vi "Perform Action.vi"(8 "error in":errorcluster, 10 "Input":variant, 11 "Thermometer DAQmx RTD Cont CFG in":refnum<class "Thermometer DAQmx RTD Cont CFG Simulated.lvclass">) -> (0 "error out":errorcluster, 2 "Output":variant, 3 "Thermometer DAQmx RTD Cont CFG out":refnum<class "Thermometer DAQmx RTD Cont CFG Simulated.lvclass">)   [LabVIEW 2024, in "DAQmx Simulated CFGs.lvlib" / "Thermometer DAQmx RTD Cont CFG Simulated.lvclass"]
uses:
  Thermometer DAQmx RTD Cont CFG Simulated.lvclass
  25f3cd8c-dbf7-49b5-a67b-aca2ec958ed2.vi
  <vilib>/JDP Science/JSONtext/Find Item.vi
  <vilib>/JDP Science/JSONtext/Next JSON Value.vi
  <vilib>/JDP Science/JSONtext/String Subset.vi
  <vilib>/JDP Science/JSONtext/Parsing/Advance past next JSON Value (inlined COPY).vi
  <vilib>/JDP Science/JSONtext/Parsing/Advance past whitespace.vi
  <vilib>/JDP Science/JSONtext/Parsing/Advance past String.vi
  <vilib>/JDP Science/JSONtext/Parsing/Advance past Number.vi
  <vilib>/JDP Science/JSONtext/Parsing/Advance past Line Ending.vi
  <vilib>/JDP Science/JSONtext/Parsing/Parse Full Path or Item Name.vi
  <vilib>/JDP Science/JSONtext/Parsing/Advance past Array.vi
  <vilib>/JDP Science/JSONtext/Parsing/Advance past Object.vi
  <vilib>/JDP Science/JSONtext/support/Error Cluster From Code.vi
  <vilib>/JDP Science/JSONtext/Offset/Find Item Locations by Path.vi
  <vilib>/JDP Science/JSONtext/JSON text to Variant.vi
  <vilib>/JDP Science/JSONtext/LVClass Serializer/JSONtext LVClass Serializer.lvclass
  Thermometer DAQmx RTD Cont CFG/Thermometer DAQmx RTD Cont CFG.lvclass
  Configurations/CFG JSON/CFG JSON.lvclass
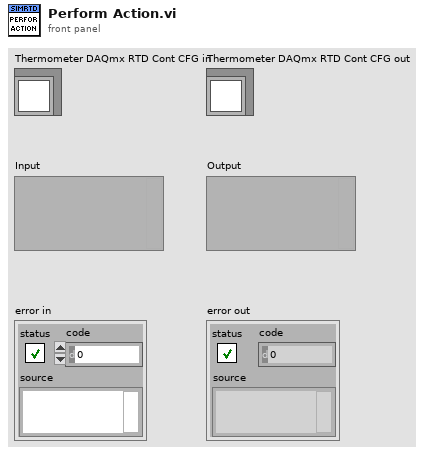
[diagram p1: front panel]
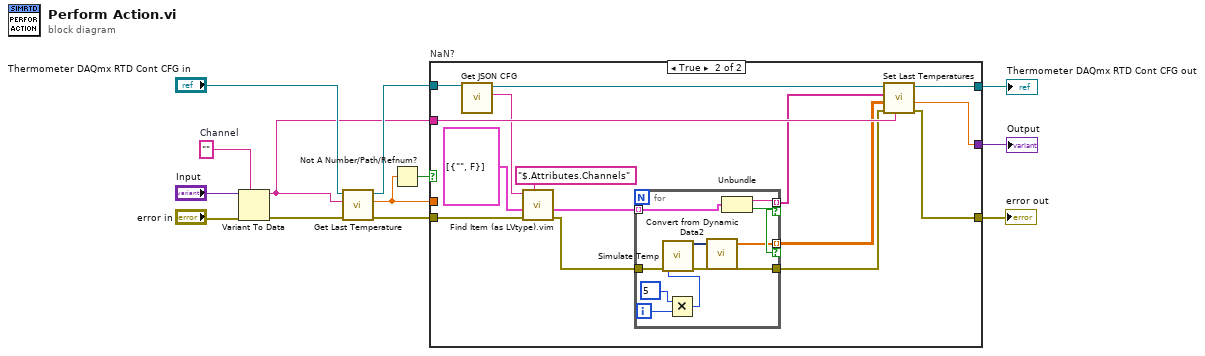
[diagram p0: block diagram]
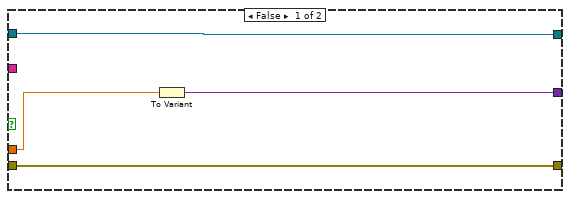
[diagram p2: hidden frame]
diagram:
  w9 = ""  # Channel
  n1 = Variant To Data(error in="error in", type=w9, Variant="Input") -> (data=w1:string, error out=w2:errorcluster)
  n2 = call "Get Last Temperature.vi"("error in"=w2, "Channel"=w1, "Thermometer DAQmx RTD Cont CFG in"="Thermometer DAQmx RTD Cont CFG in") -> ("error out"=w11:errorcluster, "Temperature"=w10:dbl, "Thermometer DAQmx RTD Cont CFG out"=w12:refnum<class "Thermometer DAQmx RTD Cont CFG Simulated.lvclass">)  [unwired: 6 in]
  n3 = Not A Number/Path/Refnum?(number/path/refnum=w10) -> (NaN/Path/Refnum?=w13:bool)
  n4 = case "NaN?" shown="True" w13 {
    tunnel: w12 -> [w15 w28]
    tunnel: w11 -> [w14 w26]
    tunnel: [w14 w32] -> w3
    tunnel: [w16 w29] -> w4
    tunnel: [w15 w31] -> w5
    tunnel: w10 -> [w17 _]
    tunnel: w1 -> [_ w30]
    frame False {
      n5 = To Variant(anything=w17) -> (Variant=w16:variant)
    }
    frame True {
      n6 = call "Get JSON CFG.vi"("CFG JSON in"=w28) -> ("<JSON> CFG"=w27:string, "CFG JSON out"=w21:refnum<class "Thermometer DAQmx RTD Cont CFG Simulated.lvclass">)  [unwired: 9 in]
      n7 = call "Find Item (as LVtype).vim"("$Path or Item Name"="$.Attributes.Channels", "error in (no error)"=w26, "Data Type and Default Value"=cluster{"Name":string, "Enabled":bool}[] [{"Name"="", "Enabled"=FALSE}], "JSON"=w27) -> ("error out"=w20:errorcluster, "Data"=w23:cluster{"Name":string, "Enabled":bool}[])  [unwired: 4 in, 2 out]
      n8 = for {
        tunnel: w23 -> [w42] mode=indexing
        tunnel: [w41] -> w22 mode=indexing if=w38
        tunnel: w20 -> [w40]
        tunnel: [w39] -> w19
        tunnel: [w33] -> w18 mode=indexing if=w38
        i -> [w37]
        n9 = Multiply(x=5, y=w37) -> (x*y=w35:i32)
        n10 = call "Simulate Temp"("Phase"=w35, "error in (no error)"=w40) -> ("Sine Temp 50-60"=w34:dynamicdata, "error out"=w39:errorcluster)  [unwired: 12 in]
        n11 = call "Convert from Dynamic Data2"("Dynamic Data Type"=w34) -> ("Array"=w33:dbl[])  [unwired: 3 in]
        n12 = Unbundle(w42) -> ("Name"=w41:string, "Enabled"=w38:bool)
      }
      n13 = call "Set Last Temperatures.vi"("Read Channel Ident"=w30, "error in"=w19, "Temperatures"=w18, "Channel Idents"=w22, "Thermometer DAQmx RTD Cont CFG in"=w21) -> ("error out"=w32:errorcluster, "Temperature"=w29:dbl, "Thermometer DAQmx RTD Cont CFG out"=w31:refnum<class "Thermometer DAQmx RTD Cont CFG Simulated.lvclass">)  [unwired: 4 in]
    }
  }
  "error out" <- w3
  "Thermometer DAQmx RTD Cont CFG out" <- w5
  "Output" <- w4
